vi "Interpreter Core.vi"(11 "Data In":T1) -> (3 "Data Out":T1)   [LabVIEW 2019]
uses:
  BrainFuck App Data.ctl
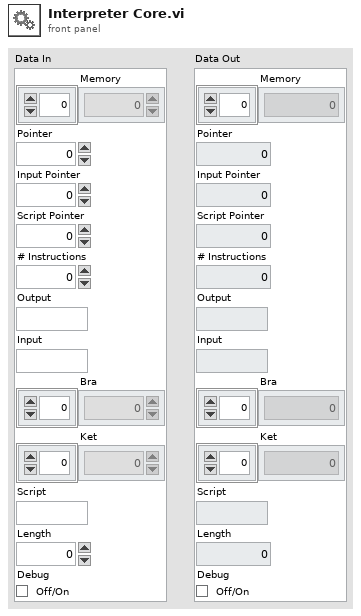
[diagram p1: front panel]
types:
  T1 = typedef "BrainFuck App Data.ctl" = cluster{"Memory":u16[], "Pointer":u64, "Input Pointer":u64, "Script Pointer":u64, "# Instructions":u64, "Output":string, "Input":string, "Bra":u64[], "Ket":u64[], "Script":string, "Length":i32, "Debug":bool}
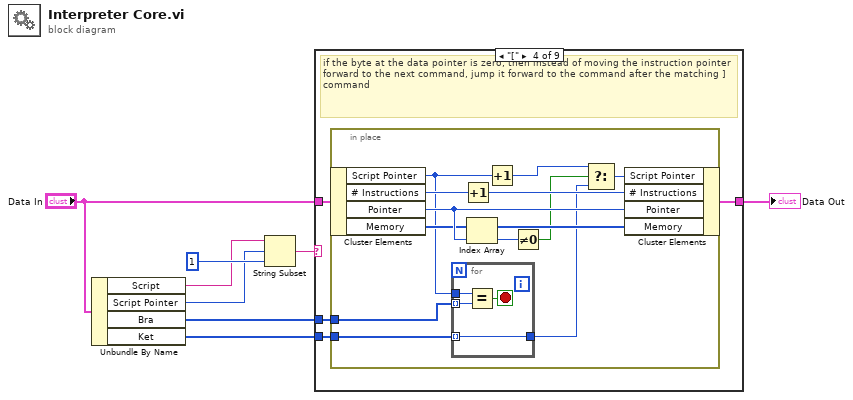
[diagram p0: block diagram]
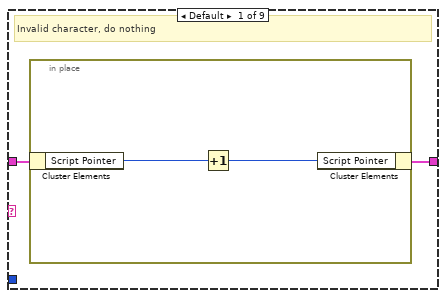
[diagram p2: hidden frame]
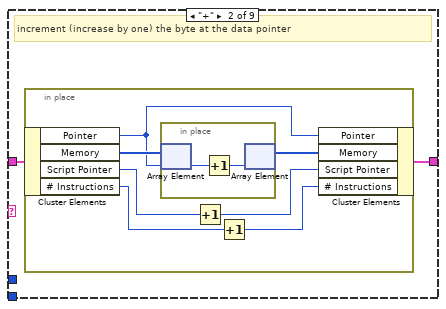
[diagram p3: hidden frame]
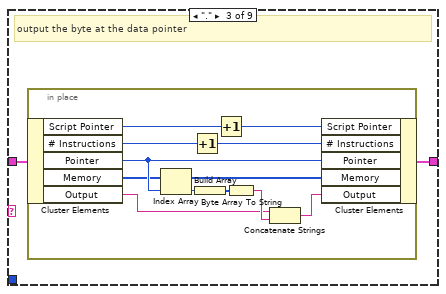
[diagram p4: hidden frame]
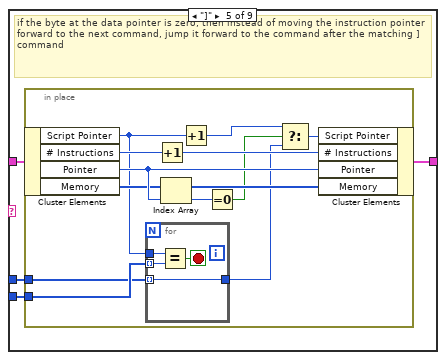
[diagram p5: hidden frame]
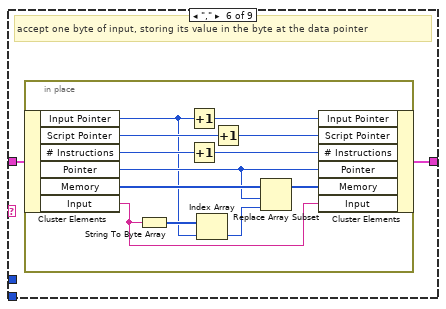
[diagram p6: hidden frame]
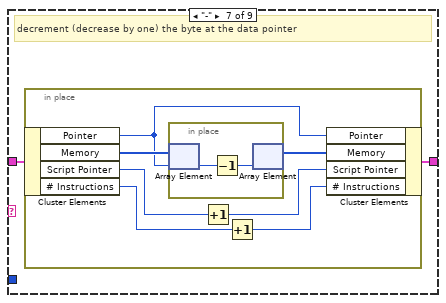
[diagram p7: hidden frame]
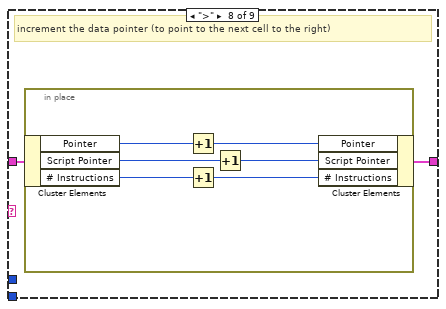
[diagram p8: hidden frame]
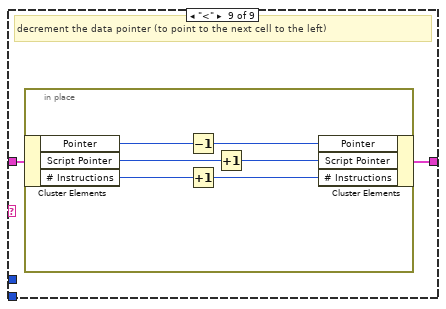
[diagram p9: hidden frame]
diagram:
  n1 = Unbundle By Name("Data In") -> ("Script"=w3:string, "Script Pointer"=w2:u64, "Bra"=w6:u64[], "Ket"=w5:u64[])
  n2 = String Subset(string=w3, offset (0)=w2, length (rest)=1 ("length (rest)")) -> (substring=w1:string)
  n3 = case shown="\"[\"" w1 {
    tunnel: "Data In" -> [w10 w14 w25 w40 w60 w78 w92 w103 w111]
    tunnel: [w9 w13 w24 w39 w59 w77 w91 w102 w110] -> w8
    tunnel: w6 -> [_ _ _ w37 w58 _ _ _ _]
    tunnel: w5 -> [_ _ _ w38 w57 _ _ _ _]
    frame Default {
      # "Invalid character, do nothing"
      n4 = in-place {
        n5 = in-place-cluster #1(w10) -> ("Script Pointer"=w12:u64)
        n6 = Increment(x=w12) -> (x+1=w11:u64)
        n7 = in-place-cluster #1("Script Pointer"=w11) -> (w9:T1)
      }
    }
    frame "+" {
      # "increment (increase by one) the byte at the data pointer"
      n8 = in-place {
        n9 = in-place-cluster #2(w14) -> ("Pointer"=w19:u64, "Memory"=w21:u16[], "Script Pointer"=w18:u64, "# Instructions"=w16:u64)
        n10 = in-place {
          n11 = in-place-array #3(w21, w19) -> (w23:u16)
          n12 = Increment(x=w23) -> (x+1=w22:u16)
          n13 = in-place-array #3(w22) -> (w20:u16[])  [unwired: 1 out]
        }
        n14 = Increment(x=w18) -> (x+1=w17:u64)
        n15 = Increment(x=w16) -> (x+1=w15:u64)
        n16 = in-place-cluster #2("Pointer"=w19, "Memory"=w20, "Script Pointer"=w17, "# Instructions"=w15) -> (w13:T1)
      }
    }
    frame "." {
      # "output the byte at the data pointer"
      n17 = in-place {
        n18 = in-place-cluster #4(w25) -> ("Script Pointer"=w32:u64, "# Instructions"=w34:u64, "Pointer"=w36:u64, "Memory"=w35:u16[], "Output"=w27:string)
        n19 = Index Array(array=w35, index=w36) -> (element=w29:u16)
        n20 = Increment(x=w34) -> (x+1=w33:u64)
        n21 = Build Array(w29) -> (w28:u16[])
        n22 = Increment(x=w32) -> (x+1=w31:u64)
        n23 = Byte Array To String(unsigned byte array=w28) -> (string=w30:string)
        n24 = Concatenate Strings(w27, w30) -> (w26:string)
        n25 = in-place-cluster #4("Script Pointer"=w31, "# Instructions"=w33, "Pointer"=w36, "Memory"=w35, "Output"=w26) -> (w24:T1)
      }
    }
    frame "[" {
      # "if the byte at the data pointer is zero, then instead of moving the instruction pointer forward to the next command, jump it forward to the command after the matching ] command"
      n26 = in-place {
        in-place-border: w38 -> [w42]
        in-place-border: w37 -> [w41]
        n27 = in-place-cluster #5(w40) -> ("Script Pointer"=w45:u64, "# Instructions"=w50:u64, "Pointer"=w52:u64, "Memory"=w51:u16[])
        n28 = for {
          tunnel: w45 -> [w56]
          tunnel: [w54] -> w44
          tunnel: w42 -> [w54] mode=indexing
          tunnel: w41 -> [w53] mode=indexing
          stop <- w55 stop-if-true
          n29 = Equal?(x=w56, y=w53) -> (x = y?=w55:bool)
        }
        n30 = Increment(x=w50) -> (x+1=w49:u64)
        n31 = Index Array(array=w51, index=w52) -> (element=w48:u16)
        n32 = Increment(x=w45) -> (x+1=w47:u64)
        n33 = Not Equal To 0?(x=w48) -> (x != 0?=w46:bool)
        n34 = Select(t=w47, s=w46, f=w44) -> (s? t:f=w43:u64)
        n35 = in-place-cluster #5("Script Pointer"=w43, "# Instructions"=w49, "Pointer"=w52, "Memory"=w51) -> (w39:T1)
      }
    }
    frame "]" {
      # "if the byte at the data pointer is zero, then instead of moving the instruction pointer forward to the next command, jump it forward to the command after the matching ] command"
      n36 = in-place {
        in-place-border: w58 -> [w61]
        in-place-border: w57 -> [w62]
        n37 = in-place-cluster #6(w60) -> ("Script Pointer"=w65:u64, "# Instructions"=w70:u64, "Pointer"=w72:u64, "Memory"=w71:u16[])
        n38 = for {
          tunnel: w65 -> [w76]
          tunnel: [w73] -> w64
          tunnel: w62 -> [w74] mode=indexing
          tunnel: w61 -> [w73] mode=indexing
          stop <- w75 stop-if-true
          n39 = Equal?(x=w76, y=w74) -> (x = y?=w75:bool)
        }
        n40 = Increment(x=w70) -> (x+1=w69:u64)
        n41 = Index Array(array=w71, index=w72) -> (element=w68:u16)
        n42 = Increment(x=w65) -> (x+1=w67:u64)
        n43 = Equal To 0?(x=w68) -> (x = 0?=w66:bool)
        n44 = Select(t=w67, s=w66, f=w64) -> (s? t:f=w63:u64)
        n45 = in-place-cluster #6("Script Pointer"=w63, "# Instructions"=w69, "Pointer"=w72, "Memory"=w71) -> (w59:T1)
      }
    }
    frame "," {
      # "accept one byte of input, storing its value in the byte at the data pointer"
      n46 = in-place {
        n47 = in-place-cluster #7(w78) -> ("Input Pointer"=w81:u64, "Script Pointer"=w87:u64, "# Instructions"=w89:u64, "Pointer"=w84:u64, "Memory"=w90:u16[], "Input"=w79:string)
        n48 = String To Byte Array(string=w79) -> (unsigned byte array=w82:u8[])
        n49 = Increment(x=w81) -> (x+1=w83:u64)
        n50 = Increment(x=w89) -> (x+1=w88:u64)
        n51 = Index Array(array=w82, index=w81) -> (element=w80:u8)
        n52 = Increment(x=w87) -> (x+1=w86:u64)
        n53 = Replace Array Subset(array=w90, new element=w80, index=w84) -> (w85:u16[])
        n54 = in-place-cluster #7("Input Pointer"=w83, "Script Pointer"=w86, "# Instructions"=w88, "Pointer"=w84, "Memory"=w85, "Input"=w79) -> (w77:T1)
      }
    }
    frame "-" {
      # "decrement (decrease by one) the byte at the data pointer"
      n55 = in-place {
        n56 = in-place-cluster #8(w92) -> ("Pointer"=w97:u64, "Memory"=w99:u16[], "Script Pointer"=w96:u64, "# Instructions"=w94:u64)
        n57 = in-place {
          n58 = in-place-array #9(w99, w97) -> (w101:u16)
          n59 = Decrement(x=w101) -> (x-1=w100:u16)
          n60 = in-place-array #9(w100) -> (w98:u16[])  [unwired: 1 out]
        }
        n61 = Increment(x=w96) -> (x+1=w95:u64)
        n62 = Increment(x=w94) -> (x+1=w93:u64)
        n63 = in-place-cluster #8("Pointer"=w97, "Memory"=w98, "Script Pointer"=w95, "# Instructions"=w93) -> (w91:T1)
      }
    }
    frame ">" {
      # "increment the data pointer (to point to the next cell to the right)"
      n64 = in-place {
        n65 = in-place-cluster #10(w103) -> ("Pointer"=w109:u64, "Script Pointer"=w108:u64, "# Instructions"=w106:u64)
        n66 = Increment(x=w109) -> (x+1=w104:u64)
        n67 = Increment(x=w106) -> (x+1=w105:u64)
        n68 = Increment(x=w108) -> (x+1=w107:u64)
        n69 = in-place-cluster #10("Pointer"=w104, "Script Pointer"=w107, "# Instructions"=w105) -> (w102:T1)
      }
    }
    frame "<" {
      # "decrement the data pointer (to point to the next cell to the left)"
      n70 = in-place {
        n71 = in-place-cluster #11(w111) -> ("Pointer"=w117:u64, "Script Pointer"=w116:u64, "# Instructions"=w114:u64)
        n72 = Decrement(x=w117) -> (x-1=w112:u64)
        n73 = Increment(x=w114) -> (x+1=w113:u64)
        n74 = Increment(x=w116) -> (x+1=w115:u64)
        n75 = in-place-cluster #11("Pointer"=w112, "Script Pointer"=w115, "# Instructions"=w113) -> (w110:T1)
      }
    }
  }
  "Data Out" <- w8
